vi "Write to Origin.vi"(0 "Origin Project Path":path=path "", 1 "Book name":string, 2 "Sheet name":string, 3 "Folder name":path=path "", 4 "Data":dbl[][](array[numeric]), 5 "error in (no error)":errorcluster, 6 "Column name":string[](array[string]), 7 "Save and exit":bool=TRUE, 8 "Column unit":string[](array[string]), 9 "Origin visible":bool=TRUE, 10 "Column comment":string[](array[string]), 12 "Column type":i32[](array[ring]) items=["COLTYPE_NO_CHANGE"=-1, "COLTYPE_Y"=0, "COLTYPE_NONE"=1, "COLTYPE_ERROR"=2, "COLTYPE_X"=3, "COLTYPE_LABEL"=4, "COLTYPE_Z"=5, "COLTYPE_X_ERROR"=6, "COLTYPE_GROUP"=7, "COLTYPE_SUBJECT"=8]) -> (19 "error out":errorcluster)   [LabVIEW 2019]
doc: "This VI connects to Origin and writes DBL data to a sheet"
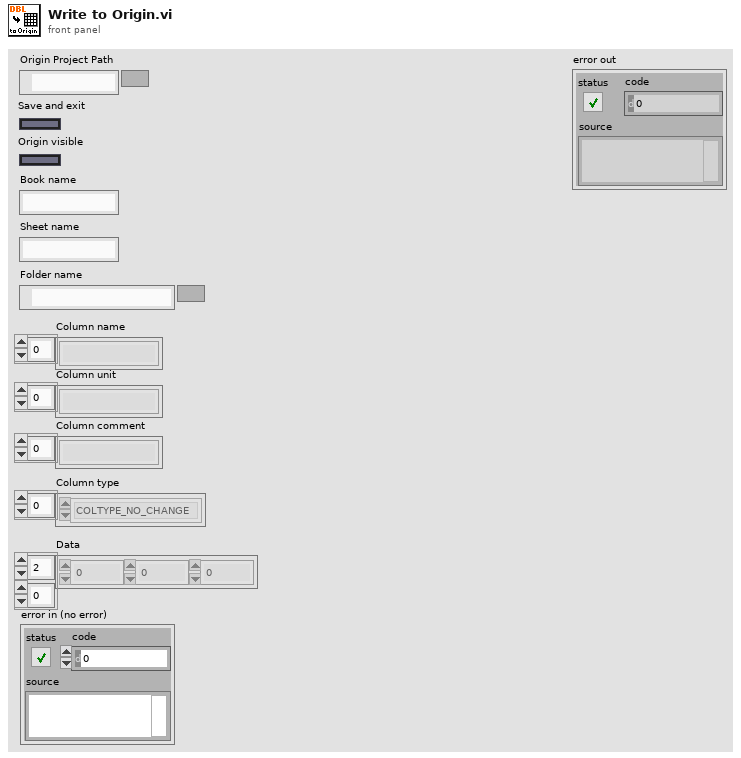
[diagram p1: front panel]
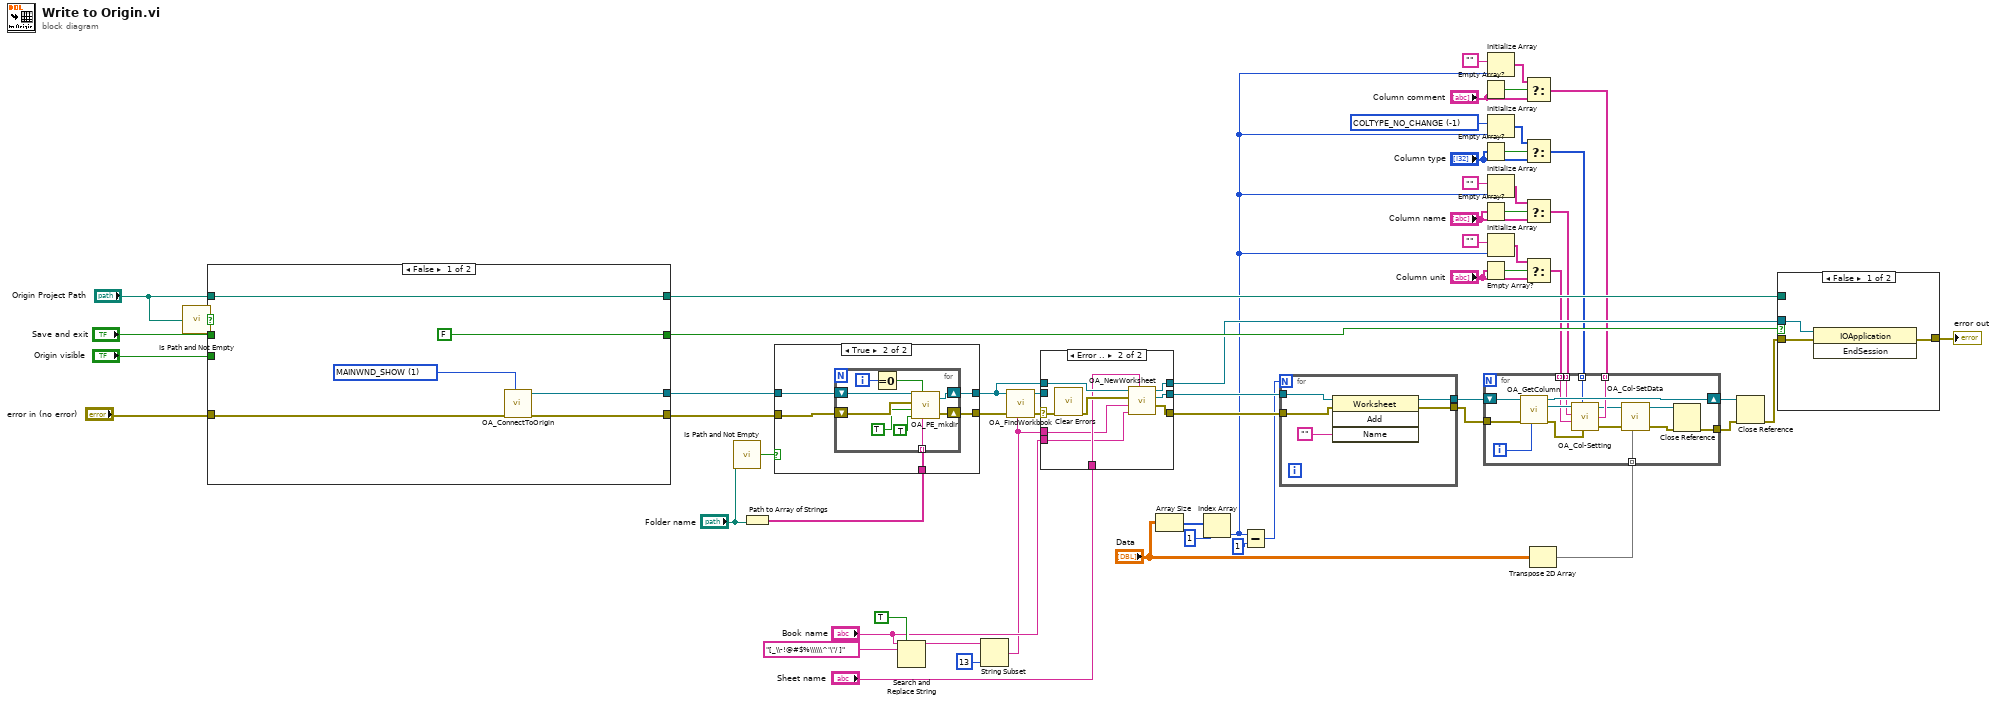
[diagram p0: block diagram]
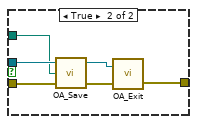
[diagram p3: hidden frame]
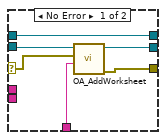
[diagram p4: hidden frame]
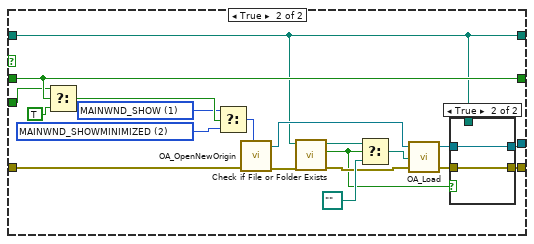
[diagram p5: hidden frame]
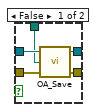
[diagram p6: hidden frame]
diagram:
  w21 = -1 items=["COLTYPE_NO_CHANGE"=-1, "COLTYPE_Y"=0, "COLTYPE_NONE"=1, "COLTYPE_ERROR"=2, "COLTYPE_X"=3, "COLTYPE_LABEL"=4, "COLTYPE_Z"=5, "COLTYPE_X_ERROR"=6, "COLTYPE_GROUP"=7, "COLTYPE_SUBJECT"=8] ("Type")
  n1 = call <vilib>:"Is Path and Not Empty.vi"("path"="Origin Project Path") -> ("Is Path and Not Empty?"=w59:bool)  [unwired: 4 in]
  n2 = case shown="False" w59 {
    tunnel: "Save and exit" -> [_ w85]
    tunnel: "Origin visible" -> [_ w84]
    tunnel: [FALSE ("Save and exit") w85] -> w42
    tunnel: "error in (no error)" -> [w64 w82]
    tunnel: [w63 w68] -> w12
    tunnel: [w62 w69] -> w13
    tunnel: "Origin Project Path" -> [w60 w67]
    tunnel: [w60 w67] -> w40
    frame False {
      w61 = 1 items=["MAINWND_HIDE"=0, "MAINWND_SHOW"=1, "MAINWND_SHOWMINIMIZED"=2, "MAINWND_SHOWMAXIMIZED"=3, "MAINWND_SHOW_BRING_TO_FRONT"=100] ("Visible")
      n3 = call <vilib>:"OA_ConnectToOrigin.vi"("Visible"=w61, "error in (no error)"=w64) -> ("error out"=w62:errorcluster, "Origin.IOApplication"=w63:refnum<k7>)  [unwired: 6 in]
    }
    frame True {
      w79 = 2 items=["MAINWND_HIDE"=0, "MAINWND_SHOW"=1, "MAINWND_SHOWMINIMIZED"=2, "MAINWND_SHOWMAXIMIZED"=3, "MAINWND_SHOW_BRING_TO_FRONT"=100] ("Visible")
      w80 = 1 items=["MAINWND_HIDE"=0, "MAINWND_SHOW"=1, "MAINWND_SHOWMINIMIZED"=2, "MAINWND_SHOWMAXIMIZED"=3, "MAINWND_SHOW_BRING_TO_FRONT"=100] ("Visible")
      n4 = Select(t=w84, s=w85, f=TRUE) -> (s? t:f=w81:bool)
      n5 = Select(t=w80, s=w81, f=w79) -> (s? t:f=w78:i32)
      n6 = call <vilib>:"OA_OpenNewOrigin.vi"("Visible"=w78, "error in (no error)"=w82) -> ("error out"=w77:errorcluster, "Origin.IOApplication dup"=w72:refnum<k7>)  [unwired: 6 in]
      n7 = call <vilib>:"Check if File or Folder Exists.vi"("error in (no error)"=w77, "path"=w67) -> ("error out"=w74:errorcluster, "file or folder exists?"=w66:bool, "dup path"=w76:path)  [unwired: 7 in]
      n8 = Select(t=w76, s=w66, f=path "" ("Path")) -> (s? t:f=w73:path)
      n9 = call <vilib>:"OA_Load.vi"("error in (no error)"=w74, "Path"=w73, "Origin.IOApplication"=w72) -> ("error out"=w70:errorcluster, "Origin.IOApplication"=w71:refnum<k7>)  [unwired: 1 out]
      n10 = case shown="True" w66 {
        tunnel: w71 -> [w90 w92]
        tunnel: w70 -> [w89 w91]
        tunnel: [w88 w91] -> w69
        tunnel: [w87 w92] -> w68
        tunnel: w67 -> [w86 _]
        frame False {
          n11 = call <vilib>:"OA_Save.vi"("Error IO"=w89, "Path"=w86, "Origin.IOApplication"=w90) -> ("Error IO Out"=w88:errorcluster, "Origin.IOApplication"=w87:refnum<k7>)  [unwired: 1 out]
        }
        frame True {
        }
      }
    }
  }
  n12 = call <vilib>:"Is Path and Not Empty.vi"("path"="Folder name") -> ("Is Path and Not Empty?"=w9:bool)  [unwired: 4 in]
  n13 = Path to Array of Strings(0:"Folder name") -> (2:w7:string[])  [unwired: 1 out]
  n14 = case shown="True" w9 {
    tunnel: w13 -> [w93 w99]
    tunnel: w12 -> [w94 w98]
    tunnel: [w94 w97] -> w11
    tunnel: [w93 w96] -> w10
    tunnel: w7 -> [_ w95]
    frame False {
    }
    frame True {
      n15 = for {
        shift-right: [w105] -> w96
        shift-left: w99 -> [w108]
        shift-right: [w106] -> w97
        shift-left: w98 -> [w107]
        tunnel: w95 -> [w102] mode=indexing
        i -> [w101]
        n16 = Equal To 0?(x=w101) -> (x = 0?=w100:bool)
        n17 = call <vilib>:"OA_PE_mkdir.vi"("name"=w102, "from root"=w100, "cd"=TRUE, "use existing"=TRUE, "Error In"=w108, "Origin.IOApplication"=w107) -> ("Error IO Out"=w105:errorcluster, "Origin.IOApplication Out"=w106:refnum<k7>)
      }
    }
  }
  n18 = Search and Replace String(replace all?=TRUE ("replace all? (F)"), input string="Book name", search string="[_\\-!@#$%\\\\\\^'\"/ ]") -> (result string=w3:string)  [unwired: 5 in, 3 out]
  n19 = String Subset(string=w3, length (rest)=13 ("length (rest)")) -> (substring=w2:string)  [unwired: 1 in]
  n20 = call <vilib>:"OA_FindWorkbook.vi"("Book Name"=w2, "error in (no error)"=w10, "Origin.IOApplication"=w11) -> ("error out"=w54:errorcluster, "Origin.WorksheetPage Out"=w53:refnum<k7>)  [unwired: 7 in]
  n21 = case shown="Error .." w54 {
    selector: w54 -> [w114 w123]
    tunnel: w53 -> [w113 _]
    tunnel: w11 -> [w109 w121]
    tunnel: "Sheet name" -> [w112 w117]
    tunnel: [w111 w118] -> w46
    tunnel: [w110 w119] -> w45
    tunnel: [w109 w120] -> w41
    tunnel: "Book name" -> [_ w116]
    tunnel: w2 -> [_ w115]
    frame No Error {
      n22 = call <vilib>:"OA_AddWorksheet.vi"("Sheet Name"=w112, "error in (no error)"=w114, "Origin.WorksheetPage In"=w113) -> ("error out"=w111:errorcluster, "Origin.Worksheet Out"=w110:refnum<k7>)  [unwired: 6 in]
    }
    frame Error {
      n23 = call <vilib>:"Clear Errors.vi"("error in (no error)"=w123) -> ("error out"=w122:errorcluster)  [unwired: 5 in, 1 out]
      n24 = call <vilib>:"OA_NewWorksheet.vi"("Sheet Name"=w117, "Book LongName"=w116, "Book Name"=w115, "error in (no error)"=w122, "Origin.IOApplication"=w121) -> ("error out"=w118:errorcluster, "Origin.Worksheet"=w119:refnum<k7>, "Origin.IOApplication"=w120:refnum<k7>)  [unwired: 2 in]
    }
  }
  n25 = Array Size(array="Data") -> (size(s)=w49:i32[])
  n26 = Index Array(array=w49, index=1) -> (element=w14:i32)
  n27 = Subtract(x=w14, y=1) -> (x-y=w15:i32)
  n28 = for {
    N: w15 -> [_]
    tunnel: w46 -> [w127]
    tunnel: w45 -> [w128]
    tunnel: [w126] -> w44
    tunnel: [w125] -> w43
    n29 = invoke class="Worksheet" method="Add"(reference=w128, error in=w127, "Name"="") -> (reference out=w125:refnum<k7>, error out=w126:errorcluster)  [unwired: 1 in, 2 out]
  }
  n30 = Empty Array?(array="Column comment") -> (empty?=w20:bool)
  n31 = Empty Array?(array="Column type") -> (empty?=w35:bool)
  n32 = Empty Array?(array="Column name") -> (empty?=w28:bool)
  n33 = Empty Array?(array="Column unit") -> (empty?=w33:bool)
  n34 = Initialize Array("", w14) -> (w19:string[])
  n35 = Initialize Array(w21, w14) -> (w34:i32[])
  n36 = Initialize Array("", w14) -> (w27:string[])
  n37 = Initialize Array("", w14) -> (w32:string[])
  n38 = Select(t=w19, s=w20, f="Column comment") -> (s? t:f=w17:string[])
  n39 = Select(t=w34, s=w35, f="Column type") -> (s? t:f=w22:i32[])
  n40 = Select(t=w27, s=w28, f="Column name") -> (s? t:f=w25:string[])
  n41 = Select(t=w32, s=w33, f="Column unit") -> (s? t:f=w31:string[])
  n42 = Transpose 2D Array(2D array="Data") -> (transposed array=w51:dbl[][])
  n43 = for {
    shift-right: [w141] -> w39
    shift-left: w43 -> [w140]
    tunnel: w22 -> [w139] mode=indexing
    tunnel: w17 -> [w138] mode=indexing
    tunnel: w25 -> [w137] mode=indexing
    tunnel: w31 -> [w136] mode=indexing
    tunnel: w51 -> [w133] mode=indexing
    tunnel: w44 -> [w132]
    tunnel: [w129] -> w38
    i -> [w144]
    n44 = call <vilib>:"OA_GetColumn.vi"("Column Name/Index"=w144, "error in (no error)"=w132, "Origin.Worksheet"=w140) -> ("error out"=w143:errorcluster, "Origin.Column"=w142:refnum<k7>, "Origin.Worksheet"=w141:refnum<k7>)  [unwired: 6 in]
    n45 = call <vilib>:"OA_Col-Setting.vi"("Origin.Column"=w142, "Type"=w139, "LongName"=w137, "Units"=w136, "error in (no error)"=w143, "Comments"=w138) -> ("Origin.Column Out"=w134:refnum<k7>, "error out"=w135:errorcluster)  [unwired: 1 in]
    n46 = call <vilib>:"OA_Col-SetData.vi"("Origin.Column"=w134, "error in (no error)"=w135, "data"=w133) -> ("Origin.Column Out"=w131:refnum<k7>, "error out"=w130:errorcluster)  [unwired: 4 in, 1 out]
    n47 = Close Reference(reference=w131, error in (no error)=w130) -> (error out=w129:errorcluster)
  }
  n48 = Close Reference(reference=w39, error in (no error)=w38) -> (error out=w37:errorcluster)
  n49 = case shown="False" w42 {
    tunnel: w41 -> [w147 w151]
    tunnel: w37 -> [w146 w150]
    tunnel: w40 -> [_ w149]
    tunnel: [w145 w148] -> w36
    frame False {
      n50 = invoke class="IOApplication" method="EndSession"(reference=w147, error in=w146) -> (error out=w145:errorcluster)  [unwired: 1 in, 2 out]
    }
    frame True {
      n51 = call <vilib>:"OA_Save.vi"("Error IO"=w150, "Path"=w149, "Origin.IOApplication"=w151) -> ("Error IO Out"=w153:errorcluster, "Origin.IOApplication"=w152:refnum<k7>)  [unwired: 1 out]
      n52 = call <vilib>:"OA_Exit.vi"("Error IO"=w153, "Origin.IOApplication"=w152) -> ("Error IO Out"=w148:errorcluster)  [unwired: 1 out]
    }
  }
  "error out" <- w36
